vi "DO-DI Line Ordering.vi"   [LabVIEW 2020]
uses:
  <vilib>/DAQmx/create/channels.llb/DAQmx Create Channel (DO-Digital Output).vi
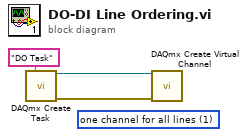
[diagram p0: block diagram]
diagram:
  (unwired) 1 items=["one channel for each line", "one channel for all lines"] ("line grouping")
  n1 = call <vilib>:"DAQmx Create Task.vi"("new task name"="DO Task" ("name to assign")) -> ("task out"=w2:refnum<k21>, "error out"=w1:errorcluster)  [unwired: 13 in]
  n2 = call-poly <vilib>:"DAQmx Create Virtual Channel.vi"("task in"=w2, "error in"=w1) -> ("lines"=w4:tag)  [unwired: 11 in, 2 out]
